vi "Distance Drive Mode.vi"(0 "Y Output High":dbl, 1 "Y Output Low":dbl, 5 "Y target":dbl, 9 "Heading target":dbl, 12 "Reinitialize":bool) -> (4 "isFinished":bool, 6 "Y out":dbl, 14 "Dist Drive Status":T1, 15 "X out":dbl)   [LabVIEW 2015]
uses:
  Common Code/Dist Drive Status.ctl
  Common Code/Change Detect Double.vi
  Robot Global Data.vi
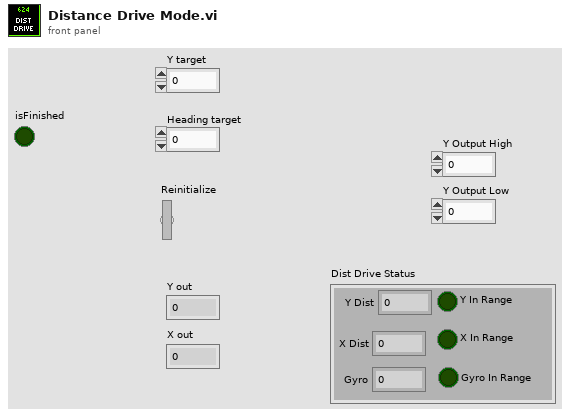
[diagram p1: front panel]
types:
  T1 = typedef "Dist Drive Status.ctl" = cluster{"Y In Range":bool, "X In Range":bool, "Gyro In Range":bool, "Y Dist":dbl, "X Dist":dbl, "Gyro":dbl}
  T2 = typedef "Dashboard Control Data.ctl" = cluster{"Shooter Presets":T3, "Encoder Control":T5, "Steer PID output":cluster{"output high":dbl, "output low":dbl}, " Steer PID gains":cluster{"proportional gain (Kc)":dbl, "integral time (Ti, min)":dbl, "derivative time (Td, min)":dbl}, "Drivetrain Settings":T6, "Vision Packet":T7, "Dashboard Drivetrain Command":T8, "Info/Command Cluster":T10, "Ball Vision Packet":T11, "Intake Presets":T13, "Intake Encoder Control":T15, "Climb Presets":T16, "Goal Output Range":cluster{"output high":dbl, "output low":dbl}, "Enabled Systems":T17, "Auton Presets":T18, "Pressure M":dbl, "Pressure B":dbl}
  T3 = typedef "Shooter Presets.ctl" = cluster{"Batter Shot":T4, "Deep Middle Shot":T4, "Manual Shot":T4, "Left Ticks Per Rotation":dbl, "Right Ticks Per Rotation":dbl, "Low Bar Shot":T4, "Shooter RPM Tolerance":dbl, "IIR Filter Power":dbl, "Trigger Power":dbl, "Fire from Load Delay":i32, "Max Angle":dbl, "Min Angle":dbl, "Angle PID gains":cluster{"P":dbl, "I":dbl, "D":dbl}, "Angle Output":cluster{"output high":dbl, "output low":dbl}, "Shooter Angle Tolerance":dbl, "Vision Shoot x^2":dbl, "Vision Shoot x":dbl, "Offset Angle":dbl, "High Goal Center Height":dbl, "Feed Forward Max Accel":dbl, "Feed Forward Kv":dbl, "Backwards Trigger":dbl, "Shot Finish Delay (ms)":dbl, "Angle Max Current":dbl, "Angle Current Trip Time":dbl, "Intake Angle":dbl, "Vision Shoot c":dbl, "Reset?":bool, "Servo Release Delay":dbl, "Servo Idle Angle":i32, "Servo Hold Angle":i32, "Angle Pot x":dbl, "Angle Pot c":dbl, "Ignore Angle?":bool, "Manual Output?":bool, "Manual Out":dbl, "Max RPM":dbl, "Safty Frist Angle":dbl, "Intake Danger Height":dbl, "Angle Pot B":i32, "Angle Pot M":dbl, "FF Finish RPM":dbl, "RPM PID Right":cluster{"P":dbl, "I":dbl, "D":dbl, "FF":dbl}, "RPM PID Left":cluster{"P":dbl, "I":dbl, "D":dbl, "FF":dbl}, "Backwards RPM":dbl, "Vision RPM":dbl}
  T4 = typedef "Shot Presets.ctl" = cluster{"Left":dbl, "Right":dbl, "Angle":dbl}
  T5 = typedef "Encoder Control.ctl" = cluster{"Right Tick Constant":dbl, "Left Tick Constant":dbl, "Reset?":bool, "Y Dist":cluster{"PID gains":cluster{"proportional gain (Kc)":dbl, "integral time (Ti, min)":dbl, "derivative time (Td, min)":dbl}}, "Y Stop Thresh":dbl, "Y Stop Speed":dbl}
  T6 = typedef "Drivetrain Settings.ctl" = cluster{"Gyro Tolerance":dbl, "Throttle Ramp (ms)":dbl, "Angular rate compensation":bool, "Throttle to Rate Scale":dbl, "Rate compensation gain":dbl, "Kv":dbl, "Ka":dbl, "Feed Forward P":dbl, "Feed Forward D":dbl, "Goal Vision PID gains":cluster{"proportional gain (Kc)":dbl, "integral time (Ti, min)":dbl, "derivative time (Td, min)":dbl}, "Goal Detection Window":dbl, "Creep Rate":dbl}
  T7 = typedef "Goal Vision Packet.ctl" = cluster{"Distance":dbl, "Center X":dbl, "Center Y":dbl, "Found Target?":bool, "Robot Center":dbl, "Angle":dbl}
  T8 = typedef "Dashboard Drivetrain Command.ctl" = cluster{"Drivetrain Vision":T9}
  T9 = typedef "Drivetrain Vision.ctl" = cluster{"Goal Window":dbl, "Ball Window":dbl}
  T10 = typedef "Ball Tracking Command Cluster.ctl" = cluster{"Distance to Ball":dbl, "Desired Angle":dbl, "Command":enum16{"Turn to Ball", "Turn to Angle", "Get Distance"}, "Pixels from Center":dbl}
  T11 = typedef "Ball Vision Packet.ctl" = cluster{"Ball Detected?":bool, "Distance to Ball":dbl, "Desired Angle":dbl, "Pixels from Center":dbl, "Tracking mode":T12}
  T12 = typedef "Tracking Mode.ctl" = enum16{"Turn to Ball", "Turn to Angle"}
  T13 = typedef "Intake Presets.ctl" = cluster{"Intake Speed":dbl, "Outake Speed":dbl, "Low Height":dbl, "Half Height":dbl, "Full Height":dbl, "Angle Speed":dbl, "Angle Tolerance":dbl, "Encoder Scale":dbl, "Load Height":dbl, "Output Range":T14, "Rotation Power Max/Min":dbl, "MaxCurrent":dbl, "Intake Trip Time":dbl, "Idle Height":dbl, "Max Height":dbl, "Reset Encoders?":bool, "PID gains":cluster{"proportional gain (Kc)":dbl, "integral time (Ti, min)":dbl, "derivative time (Td, min)":dbl}, "Intake Stop Delay":u32}
  T14 = typedef "Drivetrain Output Range.ctl" = cluster{"output high":dbl, "output low":dbl}
  T15 = typedef "IntakeEcoderControl.ctl" = cluster{"Arm Tick Constant":dbl, "Reset?":bool, "Y Dist":cluster{"PID gains":cluster{"proportional gain (Kc)":dbl, "integral time (Ti, min)":dbl, "derivative time (Td, min)":dbl}}, "Y Stop Thresh":dbl, "Y Stop Speed":dbl}
  T16 = typedef "Climb Presets.ctl" = cluster{"Pull Power":dbl, "Time to Hold":dbl, "Extend Power":dbl}
  T17 = typedef "Enabled Systems.ctl" = cluster{"Shoot":bool, "Intake":bool, "DT":bool, "Gyro":bool, "100ms":bool, "US":bool}
  T18 = typedef "Autonomous Presets.ctl" = cluster{"Pitch Limit":dbl, "Roll Limit":dbl, "Ultrasonic Limit":dbl, "Start Position":dbl, "Cross Position":dbl}
  T19 = typedef "Encoder Values Super Cluster.ctl" = cluster{"Left Encoder":T20, "Right Encoder":T20}
  T20 = typedef "Encoder Values.ctl" = cluster{"Distance":dbl, "Speed":dbl, "Ticks":dbl}
  T21 = cluster{"PID gains":cluster{"proportional gain (Kc)":dbl, "integral time (Ti, min)":dbl, "derivative time (Td, min)":dbl}}
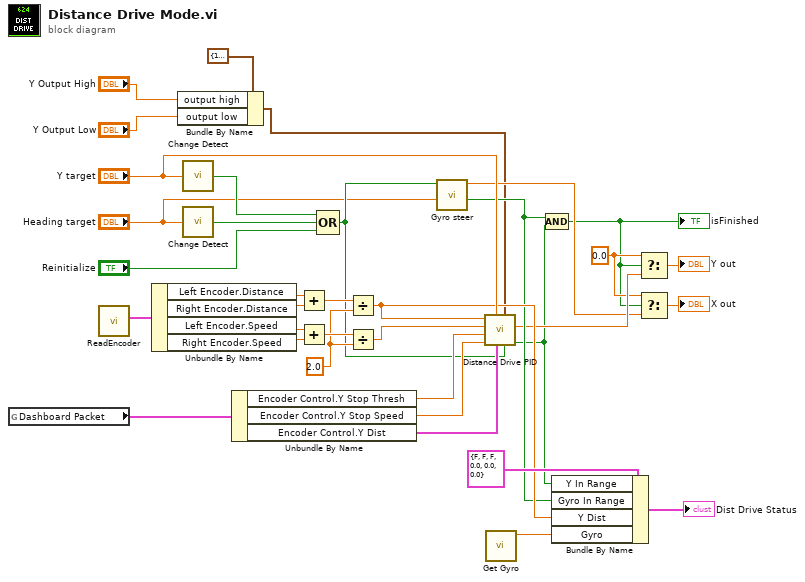
[diagram p0: block diagram]
diagram:
  w6 = 0.0 ("t")
  w25 = 2.0 ("y")
  n1 = global read "Robot Global Data.vi" "Dashboard Packet"() -> (w24:T2)
  n2 = call "ReadEncoder.vi"() -> ("Quick Use Cluster"=w22:T19)  [unwired: 11 in]
  n3 = Unbundle By Name(w22) -> ("Left Encoder.Distance"=w29:dbl, "Right Encoder.Distance"=w30:dbl, "Left Encoder.Speed"=w31:dbl, "Right Encoder.Speed"=w32:dbl)
  n4 = Bundle By Name(cluster=cluster{"output high":dbl, "output low":dbl} {"output high"=100.0, "output low"=-100.0} ("output range"), "output high"="Y Output High", "output low"="Y Output Low") -> (w1:cluster{"output high":dbl, "output low":dbl})
  n5 = call-poly "Change Detect.vi"("In"="Y target") -> ("Changed?"=w33:bool)
  n6 = call-poly "Change Detect.vi"("In"="Heading target") -> ("Changed?"=w35:bool)
  n7 = Unbundle By Name(w24) -> ("Encoder Control.Y Stop Thresh"=w21:dbl, "Encoder Control.Y Stop Speed"=w20:dbl, "Encoder Control.Y Dist"=w23:T21)
  n8 = Add(x=w29, y=w30) -> (x+y=w27:dbl)
  n9 = Add(x=w31, y=w32) -> (x+y=w28:dbl)
  n10 = Compound Arithmetic op=OR(w33, w35, "Reinitialize") -> (w16:bool)
  n11 = Divide(x=w27, y=w25) -> (x/y=w11:dbl)
  n12 = Divide(x=w28, y=w25) -> (x/y=w26:dbl)
  n13 = call "Gyro steer.vi"("Target Angle"="Heading target", "Changed?"=w16) -> ("In Range?"=w10:bool, "X out"=w5:dbl)  [unwired: 8 in]
  n14 = call "Distance Drive PID.vi"("reinitialize? (F)"=w16, "output range"=w1, "PID Params"=w23, "Setpoint"="Y target", "Max Stop Speed"=w20, "Distance Stop"=w21, "Current Speed"=w26, "Current Distance"=w11) -> ("Finished"=w3:bool, "output"=w9:dbl)  [unwired: 2 in]
  n15 = call "Get Gyro.vi"() -> ("Angle"=w12:dbl)  [unwired: 11 in]
  n16 = Compound Arithmetic op=AND(w10, w3) -> (w4:bool)
  "isFinished" <- w4
  n17 = Bundle By Name(cluster=T1 {"Y In Range"=FALSE, "X In Range"=FALSE, "Gyro In Range"=FALSE, "Y Dist"=0.0, "X Dist"=0.0, "Gyro"=0.0} ("Dist Drive Status"), "Y In Range"=w3, "Gyro In Range"=w10, "Y Dist"=w11, "Gyro"=w12) -> (→"Dist Drive Status":T1)
  n18 = Select(t=w6, s=w4, f=w9) -> (s? t:f=→"Y out":dbl)
  n19 = Select(t=w6, s=w4, f=w5) -> (s? t:f=→"X out":dbl)
